vi "Average Sectors.vi"   [LabVIEW 2013]
uses:
  <vilib>/rvi/Memory/Memory_Emulation/niFpgaMemoryEmulationReadFromVariant.vi
  <vilib>/rvi/Emulation/niFpgaSctlEmulationGetInTimedLoop.vi
  <vilib>/rvi/Memory/Memory_Emulation/niFpgaMemoryEmulationWriteToVariant.vi
  Globals/Accumulated Sector Intensity.vi
  <vilib>/rvi/DataTransferAndStorage/Container/Common/niFpgaContainerGetUniqueNameForEmu.vi
  <vilib>/rvi/errors/niFpgaSetErrorForExecOnDevCompSimple.vi
  <vilib>/rvi/Memory/Memory_Emulation/nirvimemoryFastEmulation.vi
  <vilib>/rvi/Memory/Memory_Emulation/nirvimemoryEmulation.vi
  Globals/Sector Parameter Global.vi
  <vilib>/rvi/FIFO/Fifo_Resource/nirvififoEmulationSetSize.vi
  <vilib>/rvi/eio/common/nirviEmuReportErrorAndStop.vi
  <vilib>/rvi/Emulation/niFpgaSctlEmulationFifoFullMgr.vi
  <vilib>/rvi/Emulation/niFpgaSctlEmulationResourceMgr.vi
  <vilib>/rvi/DataTransferAndStorage/Container/XNode/niFpgaContainer.xnode
  <vilib>/rvi/FIFO/Fifo_Resource/nirvififoEmulationWrite.vi
types:
  T1 = cluster{"Accumulated Intensity":fxp<+,20,20>, "Count":fxp<+,12,12>}[]
  T2 = cluster{"Accumulated Intensity":fxp<+,20,20>, "Count":fxp<+,12,12>}
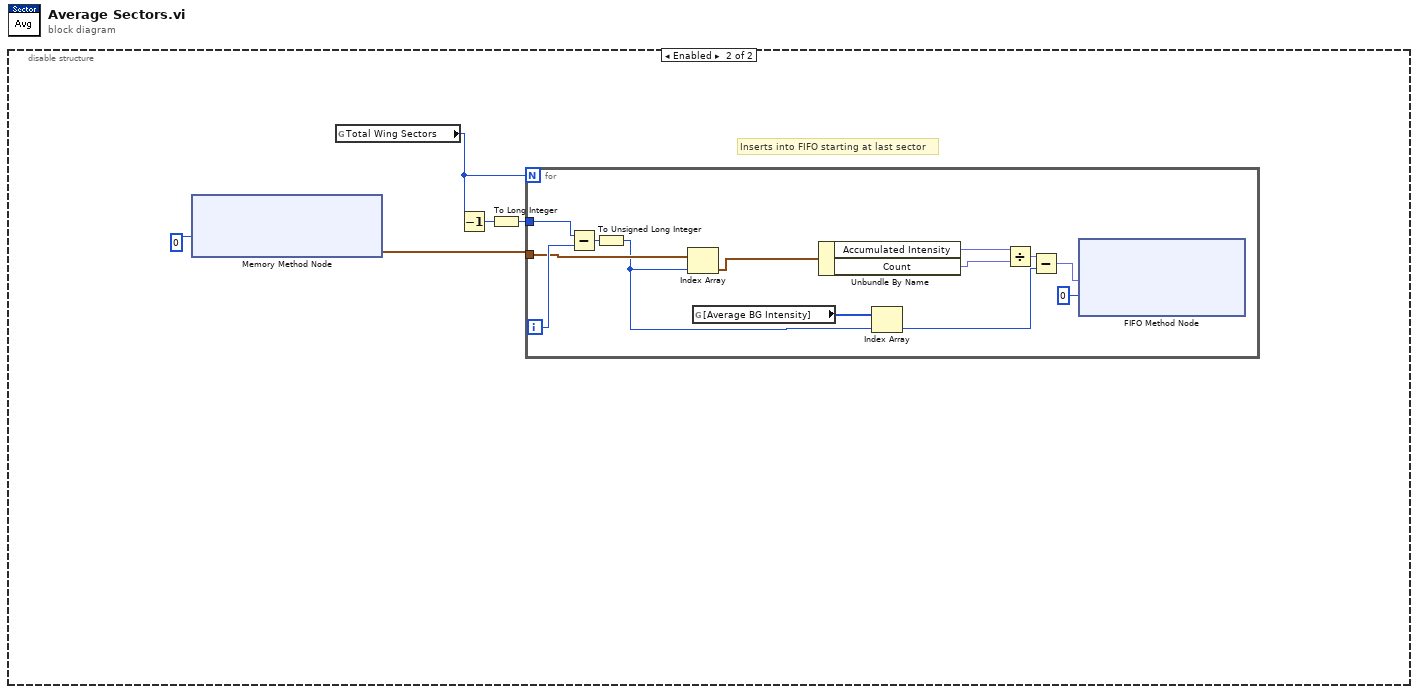
[diagram p0: block diagram]
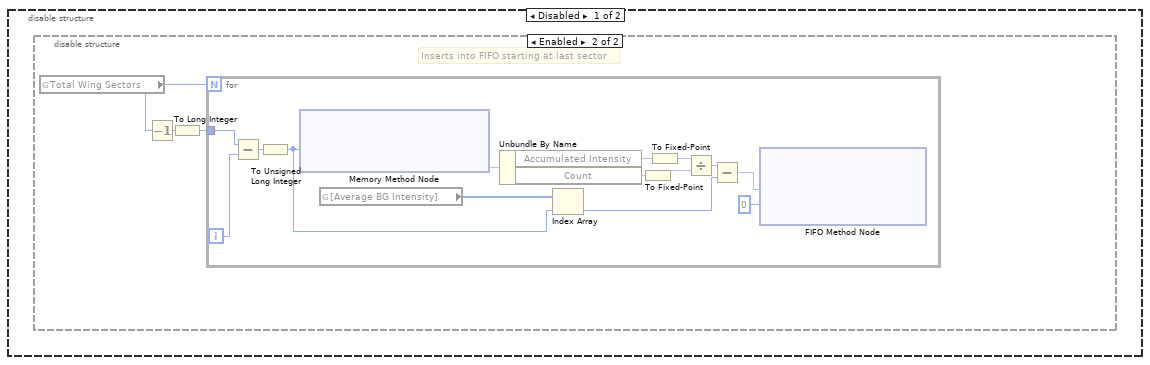
[diagram p2: hidden frame]
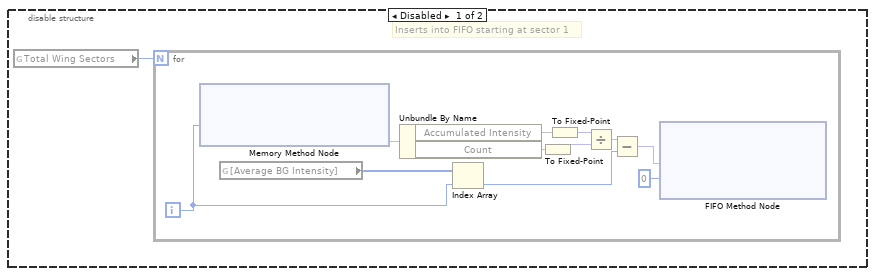
[diagram p3: hidden frame]
diagram:
  n1 = disable-structure shown="Enabled" {
    frame Disabled {
      n2 = disable-structure shown="Enabled" {
        frame Disabled {
          # "Inserts into FIFO starting at sector 1"
          n3 = global read "Accumulated Sector Intensity.vi" "Total Wing Sectors"() -> (w1:u8)
          n4 = for {
            N: w1 -> [_]
            i -> [w5]
            n5 = xnode ("Memory Method Node")("Address"=w5) -> ("Data"=w8)  [unwired: 1 in, 1 out]
            n6 = global read "Sector Parameter Global.vi" "[Average BG Intensity]"() -> (w6:u8[])
            n7 = Unbundle By Name(w8) -> ("Accumulated Intensity"=w12, "Count"=w11)
            n8 = Index Array(array=w6, index=w5) -> (element=w3:u8)
            n9 = To Fixed-Point(number=w11) -> (fixed-point=w9:fxp<+,16,16>)  [unwired: 1 in]
            n10 = To Fixed-Point(number=w12) -> (fixed-point=w10:fxp<+,32,32>)  [unwired: 1 in]
            n11 = Divide(x=w10, y=w9) -> (x/y=w4:fxp<+,8,8>)
            n12 = Subtract(x=w4, y=w3) -> (x-y=w2:fxp<+/-,9,9>)
            n13 = xnode ("FIFO Method Node")("Element"=w2, "Timeout"=0) -> ()  [unwired: 1 in, 2 out]
          }
        }
        frame Enabled {
          # "Inserts into FIFO starting at last sector"
          n14 = global read "Accumulated Sector Intensity.vi" "Total Wing Sectors"() -> (w15:u8)
          n15 = Decrement(x=w15) -> (x-1=w14:u8)
          n16 = To Long Integer(number=w14) -> (32bit integer=w13:i32)
          n17 = for {
            N: w15 -> [_]
            tunnel: w13 -> [w19]
            i -> [w17]
            n18 = Subtract(x=w19, y=w17) -> (x-y=w18:i32)
            n19 = To Unsigned Long Integer(number=w18) -> (unsigned 32bit integer=w16:u32)
            n20 = xnode ("Memory Method Node")("Address"=w16) -> ("Data"=w25)  [unwired: 1 in, 1 out]
            n21 = global read "Sector Parameter Global.vi" "[Average BG Intensity]"() -> (w23:u8[])
            n22 = Unbundle By Name(w25) -> ("Accumulated Intensity"=w29, "Count"=w28)
            n23 = Index Array(array=w23, index=w16) -> (element=w21:u8)
            n24 = To Fixed-Point(number=w28) -> (fixed-point=w26:fxp<+,16,16>)  [unwired: 1 in]
            n25 = To Fixed-Point(number=w29) -> (fixed-point=w27:fxp<+,32,32>)  [unwired: 1 in]
            n26 = Divide(x=w27, y=w26) -> (x/y=w22:fxp<+,8,8>)
            n27 = Subtract(x=w22, y=w21) -> (x-y=w20:fxp<+/-,9,9>)
            n28 = xnode ("FIFO Method Node")("Element"=w20, "Timeout"=0) -> ()  [unwired: 1 in, 2 out]
          }
        }
      }
    }
    frame Enabled {
      # "Inserts into FIFO starting at last sector"
      n29 = xnode ("Memory Method Node")("Address"=u32 0) -> ("Data"=w30:T1)  [unwired: 1 in, 1 out]
      n30 = global read "Accumulated Sector Intensity.vi" "Total Wing Sectors"() -> (w32:u8)
      n31 = Decrement(x=w32) -> (x-1=w34:u8)
      n32 = To Long Integer(number=w34) -> (32bit integer=w33:i32)
      n33 = for {
        N: w32 -> [_]
        tunnel: w33 -> [w42]
        tunnel: w30 -> [w39]
        i -> [w40]
        n34 = Subtract(x=w42, y=w40) -> (x-y=w41:i32)
        n35 = To Unsigned Long Integer(number=w41) -> (unsigned 32bit integer=w38:u32)
        n36 = Index Array(array=w39, index=w38) -> (element=w37:T2)
        n37 = global read "Sector Parameter Global.vi" "[Average BG Intensity]"() -> (w46:u8[])
        n38 = Unbundle By Name(w37) -> ("Accumulated Intensity"=w36:fxp<+,20,20>, "Count"=w35:fxp<+,12,12>)
        n39 = Index Array(array=w46, index=w38) -> (element=w44:u8)
        n40 = Divide(x=w36, y=w35) -> (x/y=w45:fxp<+,8,8>)
        n41 = Subtract(x=w45, y=w44) -> (x-y=w43:fxp<+/-,9,9>)
        n42 = xnode ("FIFO Method Node")("Element"=w43, "Timeout"=0) -> ()  [unwired: 1 in, 2 out]
      }
    }
  }
